vi "CR-导丝上料一致性检测参数读取.vi"(7 "error in (no error)":errorcluster caption="错误输入（无错误）", 10 "基路径":path) -> (0 "error out":errorcluster caption="错误输出", 1 "CR位置范围设定":T1={"位置1"={"上限"=726.0, "下限"=686.0}, "位置2"={"上限"=874.0, "下限"=834.0}, "位置3"={"上限"=997.0, "下限"=957.0}, "位置4"={"上限"=1139.0, "下限"=1099.0}, "位置5"={"上限"=1283.0, "下限"=1243.0}, "位置6"={"上限"=1429.0, "下限"=1389.0}, "位置7"={"上限"=1576.0, "下限"=1536.0}, "位置8"={"上限"=1728.0, "下限"=1688.0}, "位置9"={"上限"=1879.0, "下限"=1839.0}, "位置10"={"上限"=2036.0, "下限"=1996.0}}, 2 "导丝上料一致性基础参数":T8={"IsNorImage"=TRUE, "Exposure Values"=100289, "ImagePath"=path "C:/Users/hedongpo/Desktop/514-hdp/Alignment Assemble System/Test Picture/B/3.bmp"} caption="参数界面" {"Exposure Values" scale=0.0..200000.0}, 3 "CR导丝上料一致性参数":T7={"Rectangle"={"Left"=0, "Top"=0, "Right"=0, "Bottom"=0, "Rotation"=0.0}, "Find Straight Edge 1"={"Number of Lines"=1, "Type"=enum."First Edge Rake", "Min. Score"=10.0, "Max. Score"=1000.0, "Orientation"=0.0, "Angle Range"=45.0, "Angle Tolerance"=1.0, "Step Size"=11, "Min. SNR (db)"=0.0, "Min. Points (%)"=25.0, "Hough Iterations"=5}, "Process (Edge Detector 1)"=enum."Get All Edges", "Edge Options (Edge Detector 1)"={"Edge Polarity"=0, "Kernel Size"=9, "Width"=1, "Minimum Edge Strength"=8.0, "Interpolation Type"=enum."Bilinear Fixed", "Data Processing Method"=enum."Average"}, "Options (Find Straight Edge 1)"={"Search Direction"=0, "Edge Options"={"Edge Polarity"=0, "Kernel Size"=3, "Width"=1, "Minimum Edge Strength"=32.0, "Interpolation Type"=enum."Bilinear Fixed", "Data Processing Method"=enum."Average"}, "Show Search Area"=TRUE, "Show Search Lines"=TRUE, "Show Edges Found"=TRUE, "Show Result"=TRUE, "Search Area Color"=65280, "Search Lines Color"=255, "Edge Locations Color"=16776960, "Result Color"=16711680, "Overlay Group Name"=""}, "Parameters (Pattern Matching 1)"={"Number of Matches Requested"=1, "Minimum Match Score"=799.0, "Angle Ranges"=[{"Start Angle"=-180.0, "End Angle"=180.0}, {"Start Angle"=0.0, "End Angle"=360.0}]}, "Template File Path (Pattern Matching 1)"=path "D:/Inspect System/Source Code/Template Program/一致性模板.png"} {"Options (Find Straight Edge 1)"."Search Direction" items=["Left to Right", "Right to Left", "Top to Bottom", "Bottom to Top"]; "Options (Find Straight Edge 1)"."Edge Options"."Edge Polarity" items=["All Edges", "Rising Edges", "Falling Edges"]; "Options (Find Straight Edge 1)"."Edge Options"."Minimum Edge Strength" format="%.2f"; "Options (Find Straight Edge 1)"."Edge Options"."Width" step=2; "Options (Find Straight Edge 1)"."Edge Options"."Kernel Size" step=2; "Edge Options (Edge Detector 1)"."Edge Polarity" items=["All Edges", "Rising Edges", "Falling Edges"]; "Find Straight Edge 1"."Min. Points (%)" min=0.0 max=100.0; "Find Straight Edge 1"."Min. SNR (db)" min=0.0; "Find Straight Edge 1"."Max. Score" min=0.0 max=1024.0; "Find Straight Edge 1"."Min. Score" min=0.0 max=1024.0 step=1.0; "Rectangle"."Rotation" format="%.2f"; "Rectangle"."Left" scale=0.0..1024.0; "Rectangle"."Right" scale=0.0..1024.0})   [LabVIEW 2017]
uses:
  <vilib>/vision/Measure.llb/Straight Edge Options.ctl
  <vilib>/vision/Measure.llb/Straight Edge Process.ctl
  <vilib>/vision/Measure.llb/Edge Options.ctl
  <vilib>/vision/Measure.llb/Edge Polarity.ctl
  <vilib>/Utility/xml.llb/Read From XML File(string).vi
  Global System.vi
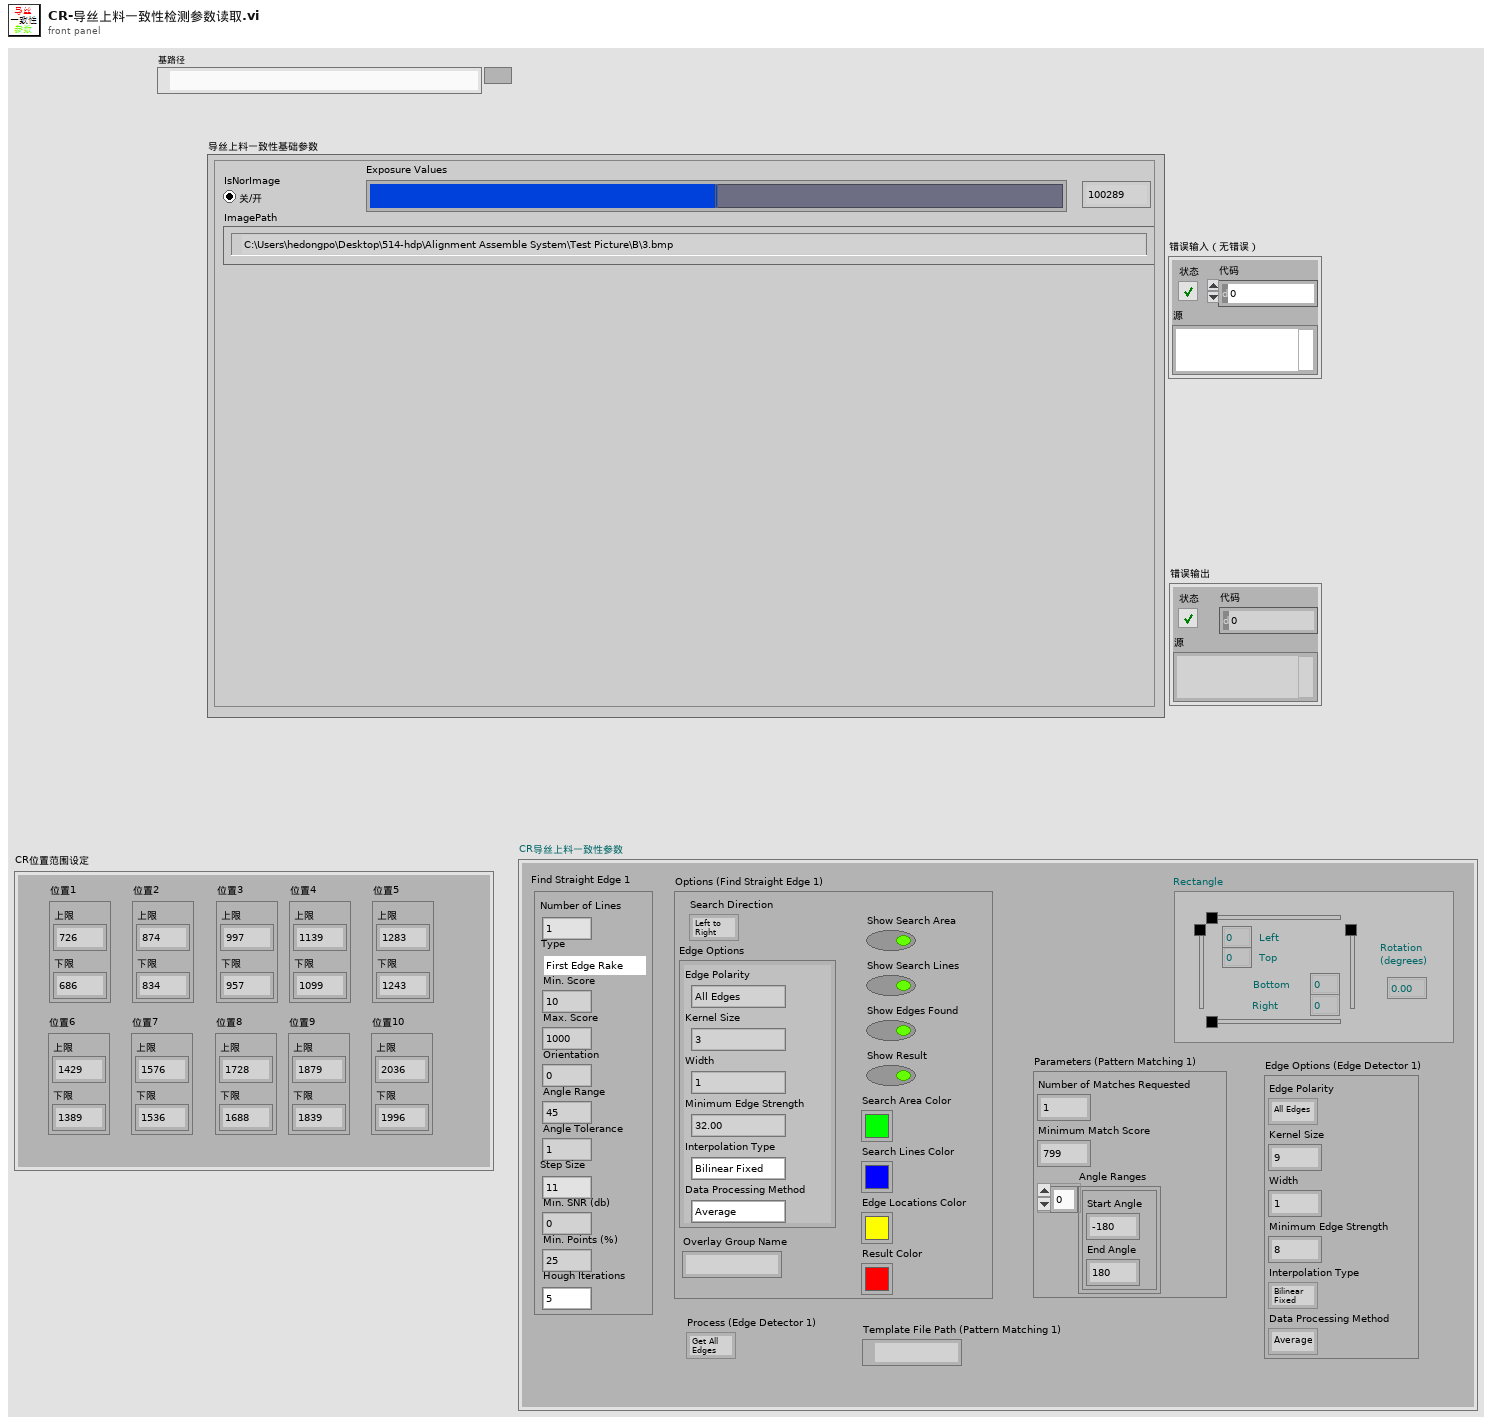
[diagram p1: front panel]
types:
  T1 = cluster{"位置1":cluster{"上限":dbl, "下限":dbl}, "位置2":cluster{"上限":dbl, "下限":dbl}, "位置3":cluster{"上限":dbl, "下限":dbl}, "位置4":cluster{"上限":dbl, "下限":dbl}, "位置5":cluster{"上限":dbl, "下限":dbl}, "位置6":cluster{"上限":dbl, "下限":dbl}, "位置7":cluster{"上限":dbl, "下限":dbl}, "位置8":cluster{"上限":dbl, "下限":dbl}, "位置9":cluster{"上限":dbl, "下限":dbl}, "位置10":cluster{"上限":dbl, "下限":dbl}}
  T2 = typedef "IMAQ Rectangle" = cluster{"Left":i32, "Top":i32, "Right":i32, "Bottom":i32, "Rotation":dbl}
  T3 = typedef "Straight Edge Options.ctl" = cluster{"Number of Lines":i32, "Type":T4, "Min. Score":dbl, "Max. Score":dbl, "Orientation":dbl, "Angle Range":dbl, "Angle Tolerance":dbl, "Step Size":u32, "Min. SNR (db)":dbl, "Min. Points (%)":dbl, "Hough Iterations":i32}
  T4 = typedef "Straight Edge Process.ctl" = enum32{"First Edge Rake", "Best Edge Rake", "Hough Edge Rake", "First Edge Projection", "Best Edge Projection"}
  T5 = typedef "Edge Options.ctl" = cluster{"Edge Polarity":T6, "Kernel Size":u32, "Width":u32, "Minimum Edge Strength":sgl, "Interpolation Type":enum32{"Zero Order", "Bilinear", "Quadratic", "Cubic", "Bilinear Fixed"}, "Data Processing Method":enum32{"Average", "Median"}}
  T6 = typedef "Edge Polarity.ctl" = u32
  T7 = cluster{"Rectangle":T2, "Find Straight Edge 1":T3, "Process (Edge Detector 1)":enum16{"Get First Edge", "Get First + Last Edge", "Get All Edges", "Get Best Edge"}, "Edge Options (Edge Detector 1)":cluster{"Edge Polarity":u32, "Kernel Size":u32, "Width":u32, "Minimum Edge Strength":sgl, "Interpolation Type":enum32{"Zero Order", "Bilinear", "Quadratic", "Cubic", "Bilinear Fixed"}, "Data Processing Method":enum32{"Average", "Median"}}, "Options (Find Straight Edge 1)":cluster{"Search Direction":u32, "Edge Options":T5, "Show Search Area":bool, "Show Search Lines":bool, "Show Edges Found":bool, "Show Result":bool, "Search Area Color":u32, "Search Lines Color":u32, "Edge Locations Color":u32, "Result Color":u32, "Overlay Group Name":string}, "Parameters (Pattern Matching 1)":cluster{"Number of Matches Requested":i32, "Minimum Match Score":sgl, "Angle Ranges":cluster{"Start Angle":sgl, "End Angle":sgl}[]}, "Template File Path (Pattern Matching 1)":path}
  T8 = cluster{"IsNorImage":bool, "Exposure Values":u32, "ImagePath":path}
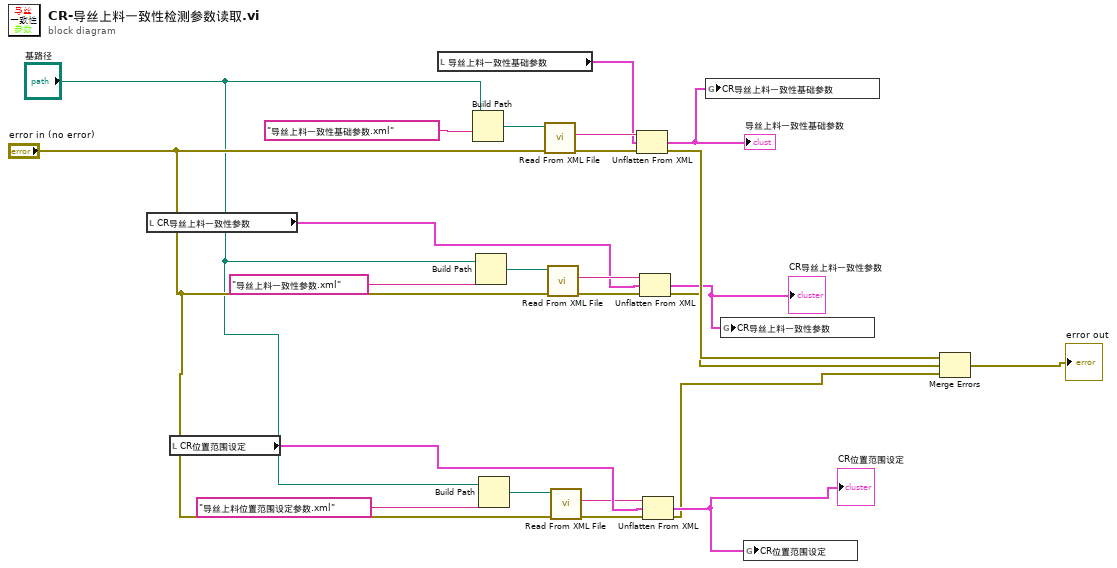
[diagram p0: block diagram]
diagram:
  n1 = local read "CR导丝上料一致性参数"() -> (w12:T7)
  n2 = local read "CR位置范围设定"() -> (w8:T1)
  n3 = local read "导丝上料一致性基础参数"() -> (w22:T8)
  n4 = Build Path(base path="基路径", name or relative path="导丝上料一致性基础参数.xml" ("名称或相对路径")) -> (appended path=w24:path)
  n5 = Build Path(base path="基路径", name or relative path="导丝上料一致性参数.xml" ("名称或相对路径")) -> (appended path=w15:path)
  n6 = Build Path(base path="基路径", name or relative path="导丝上料位置范围设定参数.xml" ("名称或相对路径")) -> (appended path=w6:path)
  n7 = call-poly <vilib>:"Read From XML File.vi"("error in (no error)"="error in (no error)", "XML File Path"=w24) -> ("error out"=w21:errorcluster, "XML Elements"=w23:string)  [unwired: 7 in, 1 out]
  n8 = call-poly <vilib>:"Read From XML File.vi"("error in (no error)"="error in (no error)", "XML File Path"=w15) -> ("error out"=w14:errorcluster, "XML Elements"=w16:string)  [unwired: 7 in, 1 out]
  n9 = call-poly <vilib>:"Read From XML File.vi"("error in (no error)"="error in (no error)", "XML File Path"=w6) -> ("error out"=w7:errorcluster, "XML Elements"=w5:string)  [unwired: 7 in, 1 out]
  n10 = Unflatten From XML(xml string=w23, type=w22, error in (no error)=w21) -> (value=w17:T8, error out=w20:errorcluster)
  "导丝上料一致性基础参数" <- w17
  n11 = Unflatten From XML(xml string=w16, type=w12, error in (no error)=w14) -> (value=w10:T7, error out=w13:errorcluster)
  "CR导丝上料一致性参数" <- w10
  n12 = Unflatten From XML(xml string=w5, type=w8, error in (no error)=w7) -> (value=w4:T1, error out=w1:errorcluster)
  "CR位置范围设定" <- w4
  n13 = global write "Global System.vi" "CR导丝上料一致性基础参数"(w17) -> ()
  n14 = global write "Global System.vi" "CR导丝上料一致性参数"(w10) -> ()
  n15 = global write "Global System.vi" "CR位置范围设定"(w4) -> ()
  n16 = Merge Errors(w20, w13, w1) -> (→"error out":errorcluster)
